vi "Energy Meter.vi"(7 "initialize":bool, 8 "error in (no error)":errorcluster, 9 "Levels":T1, 10 "Set":T2 {"PSD Filter"."Forward Coefficients" format="%.4f"; "PSD Filter"."Reverse Coefficients" format="%.4f"}, 11 "DATA IN":waveform(dbl)) -> (0 "error out":errorcluster, 3 "DATA OUT":T3)   [LabVIEW 2017, in "Processing.lvlib"]
uses:
  Processing.lvlib
  Energy Meter Data OUT.ctl
  Filters.ctl
  Levels.ctl
  <vilib>/ptbypt/NI_PtbyPt.lvlib
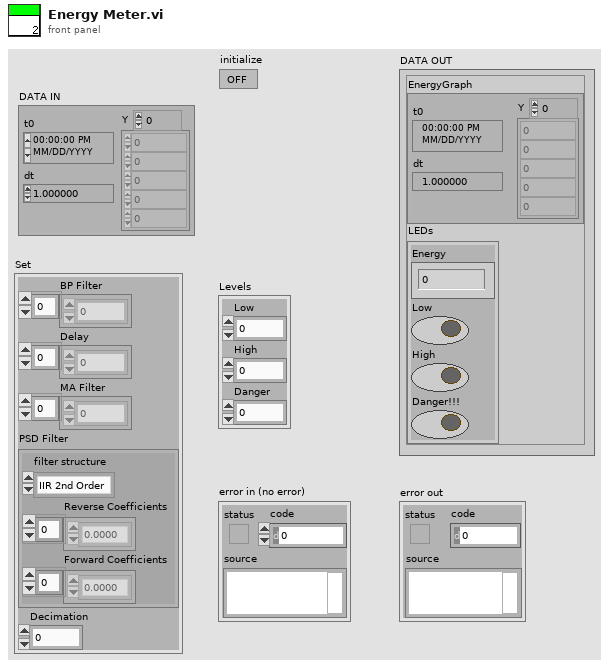
[diagram p1: front panel]
types:
  T1 = typedef "Processing.lvlib/Levels.ctl" = cluster{"Low":i32, "High":i32, "Danger":i32}
  T2 = typedef "Processing.lvlib/Filters.ctl" = cluster{"BP Filter":dbl[], "Delay":dbl[], "MA Filter":dbl[], "PSD Filter":cluster{"filter structure":enum32{"IIR 2nd Order", "IIR 4th Order"}, "Reverse Coefficients":dbl[], "Forward Coefficients":dbl[]}, "Decimation":i32}
  T3 = typedef "Processing.lvlib/Energy Meter Data OUT.ctl" = cluster{"EnergyGraph":waveform(dbl), "LEDs":cluster{"Energy":dbl, "Low":bool, "High":bool, "Danger!!!":bool}}
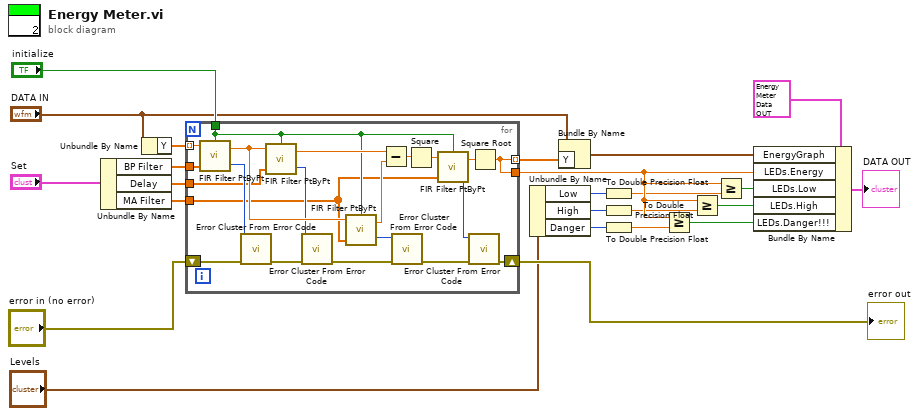
[diagram p0: block diagram]
diagram:
  n1 = Unbundle By Name("Set") -> ("BP Filter"=w18:dbl[], "Delay"=w17:dbl[], "MA Filter"=w16:dbl[])
  n2 = Unbundle By Name("DATA IN") -> ("Y"=w5:dbl[])
  n3 = for {
    tunnel: "initialize" -> [w38]
    tunnel: w18 -> [w29]
    tunnel: w17 -> [w28]
    tunnel: w16 -> [w27]
    shift-right: [w31] -> w21
    shift-left: "error in (no error)" -> [w30]
    tunnel: [w25] -> w6 mode=indexing
    tunnel: w5 -> [w26] mode=indexing
    tunnel: [w25] -> w15
    n4 = call <vilib>:"FIR Filter PtByPt.vi"("initialize"=w38, "Forward Coefficients"=w29, "x"=w26) -> ("error"=w39:i32, "Filtered x"=w45:dbl)  [unwired: 1 in]
    n5 = call <vilib>:"Error Cluster From Error Code.vi"("error in (no error)"=w30, "error code (0)"=w39) -> ("error out"=w34:errorcluster)  [unwired: 7 in]
    n6 = call <vilib>:"FIR Filter PtByPt.vi"("initialize"=w38, "Forward Coefficients"=w28, "x"=w45) -> ("error"=w37:i32, "Filtered x"=w44:dbl)  [unwired: 1 in]
    n7 = call <vilib>:"Error Cluster From Error Code.vi"("error in (no error)"=w34, "error code (0)"=w37) -> ("error out"=w33:errorcluster)  [unwired: 7 in]
    n8 = call <vilib>:"FIR Filter PtByPt.vi"("initialize"=w38, "Forward Coefficients"=w27, "x"=w45) -> ("error"=w36:i32, "Filtered x"=w43:dbl)  [unwired: 1 in]
    n9 = Subtract(x=w44, y=w43) -> (x-y=w42:dbl)
    n10 = call <vilib>:"Error Cluster From Error Code.vi"("error in (no error)"=w33, "error code (0)"=w36) -> ("error out"=w32:errorcluster)  [unwired: 7 in]
    n11 = Square(x=w42) -> (x^2=w41:dbl)
    n12 = call <vilib>:"FIR Filter PtByPt.vi"("initialize"=w38, "Forward Coefficients"=w27, "x"=w41) -> ("error"=w35:i32, "Filtered x"=w40:dbl)  [unwired: 1 in]
    n13 = call <vilib>:"Error Cluster From Error Code.vi"("error in (no error)"=w32, "error code (0)"=w35) -> ("error out"=w31:errorcluster)  [unwired: 7 in]
    n14 = Square Root(x=w40) -> (sqrt(x)=w25:dbl)
  }
  "error out" <- w21
  n15 = Unbundle By Name("Levels") -> ("Low"=w10:i32, "High"=w9:i32, "Danger"=w8:i32)
  n16 = Bundle By Name(cluster="DATA IN", "Y"=w6) -> (w7:waveform(dbl))
  n17 = To Double Precision Float(number=w10) -> (double precision float=w3:dbl)
  n18 = To Double Precision Float(number=w9) -> (double precision float=w2:dbl)
  n19 = To Double Precision Float(number=w8) -> (double precision float=w1:dbl)
  n20 = Greater Or Equal?(x=w15, y=w1) -> (x >= y?=w14:bool)
  n21 = Greater Or Equal?(x=w15, y=w2) -> (x >= y?=w13:bool)
  n22 = Greater Or Equal?(x=w15, y=w3) -> (x >= y?=w12:bool)
  n23 = Bundle By Name(cluster=T3 {"EnergyGraph"={"t0"=timestamp(0 s since 1904-01-01), "dt"=1.0, "Y"=[]}, "LEDs"={"Energy"=0.0, "Low"=FALSE, "High"=FALSE, "Danger!!!"=FALSE}} ("input cluster"), "EnergyGraph"=w7, "LEDs.Energy"=w15, "LEDs.Low"=w12, "LEDs.High"=w13, "LEDs.Danger!!!"=w14) -> (→"DATA OUT":T3)
